vi "rqcAlice PM Level Test (Low Level Example).vi"() -> ()   [LabVIEW 2019]
uses:
  FPGA/Alice/Custom Controls/Main State Machine/rqcAlice DAC Clock Positions.ctl
  Shared/Shared FPGA Lib/Shared Logic/Custom Controls/rqc Random Generator.parameters.ctl
  Shared/Shared FPGA Lib/Shared Logic/Custom Controls/rqc Random Generator.value type.ctl
  FPGA/Alice/Custom Controls/Phase Modulator/rqcAlice Mod.Config.ctl
  Custom Controls/rqcAlice States.ctl
  Shared/Shared Host Lib/rqc ServiceNET/Custom Controls/rqc ServiceNET command.ctl
  Shared/Shared Host Lib/rqc ServiceNET/Alice/Custom Controls/rqcAlice ServiceNET control.ctl
  <vilib>/FPGAPlugInAG/PCIe-7820R/niLvFpga_Open_PCIe-7820R.vi
  <vilib>/rvi/interface/common/dynamic/niFpgaDynamicAddResources.vi
  <vilib>/FPGAPlugInAG/Dynamic/niLvFpga_Close_Dynamic.vi
  <vilib>/rvi/interface/nirviOpenFPGA/nirviOpenFPGA.xnode
  FPGA Bitfiles/rqcAlice FPGA (7820R) v 3.2.0.lvbitx
  <vilib>/rvi/interface/nirviCloseFPGA/nirviCloseFPGA.xnode
panel:
  in  "Tab Control":enum32{"Alice PM config", "Advanced parameters"}(tab)
  in  "Sync mode":bool caption="«Coax / SD»"
  in  "PM.DAC parameters":T1={"value type"=enum."constant", "constant"=512, "num of levels"=4, "levels values"=[512, 512, 512, 512]} caption="Phase modulation value" {"num of levels" min=4 max=4 step=1}
  in  "PM min":u16
  in  "PM max":u16=512
  in  "PM increment":u16=8
  out "PM value scanned":u16=512
  in  "Delay line value":u32
  in  "Modulator config":T3={"mod.on"=9, "mod.off"=1}
  in  "DAC Clock params":T4=[18, 38]
  out "IP Address":string="10.32.64.203"
  out "Num of Detections vs DAC Level":T5(graph)={"appended array"=[0.0, 8.0, 16.0, 24.0, 32.0, 40.0, 48.0, 56.0, 64.0, 72.0, 80.0, 88.0, 96.0, 104.0, 112.0, 120.0, 128.0, 136.0, 144.0, 152.0, 160.0, 168.0, 176.0, 184.0, 192.0, 200.0, 208.0, 216.0, 224.0, 232.0, 240.0, 248.0, 256.0, 264.0, 272.0, 280.0, 288.0, 296.0, 304.0, 312.0, 320.0, 328.0, 336.0, 344.0, 352.0, 360.0, 368.0, 376.0, 384.0, 392.0, 400.0, 408.0, 416.0, 424.0, 432.0, 440.0, 448.0, 456.0, 464.0, 472.0, 480.0, 488.0, 496.0, 504.0, 512.0, 512.0], "appended array"=[0.0, 0.0, 0.0, 0.0, 0.0, 0.0, 0.0, 0.0, 0.0, 0.0, 0.0, 0.0, 0.0, 0.0, 0.0, 0.0, 0.0, 0.0, 0.0, 0.0, 0.0, 0.0, 0.0, 0.0, 0.0, 0.0, 0.0, 0.0, 0.0, 0.0, 0.0, 0.0, 0.0, 0.0, 0.0, 0.0, 0.0, 0.0, 0.0, 0.0, 0.0, 0.0, 0.0, 0.0, 0.0, 0.0, 0.0, 0.0, 0.0, 0.0, 0.0, 0.0, 0.0, 0.0, 0.0, 0.0, 0.0, 0.0, 0.0, 0.0, 0.0, 0.0, 0.0, 0.0, 0.0]}
  out "error out":errorcluster
  in  "Stop":bool
  out "Connection status":bool
  in  "port":u16=5020
  out "Current State":T6=enum."App.Stop" caption="App current state"
  in  "Attenuation, dB":dbl=10.0 max=40.0
  # "LAN settings:"
  # "«"
  # "»"
  # "Constant"
  # "Random"
  # "Recommended [18]\n[38]"
  # "Recommended mod.on - [9]\nmod.off - [1-2]"
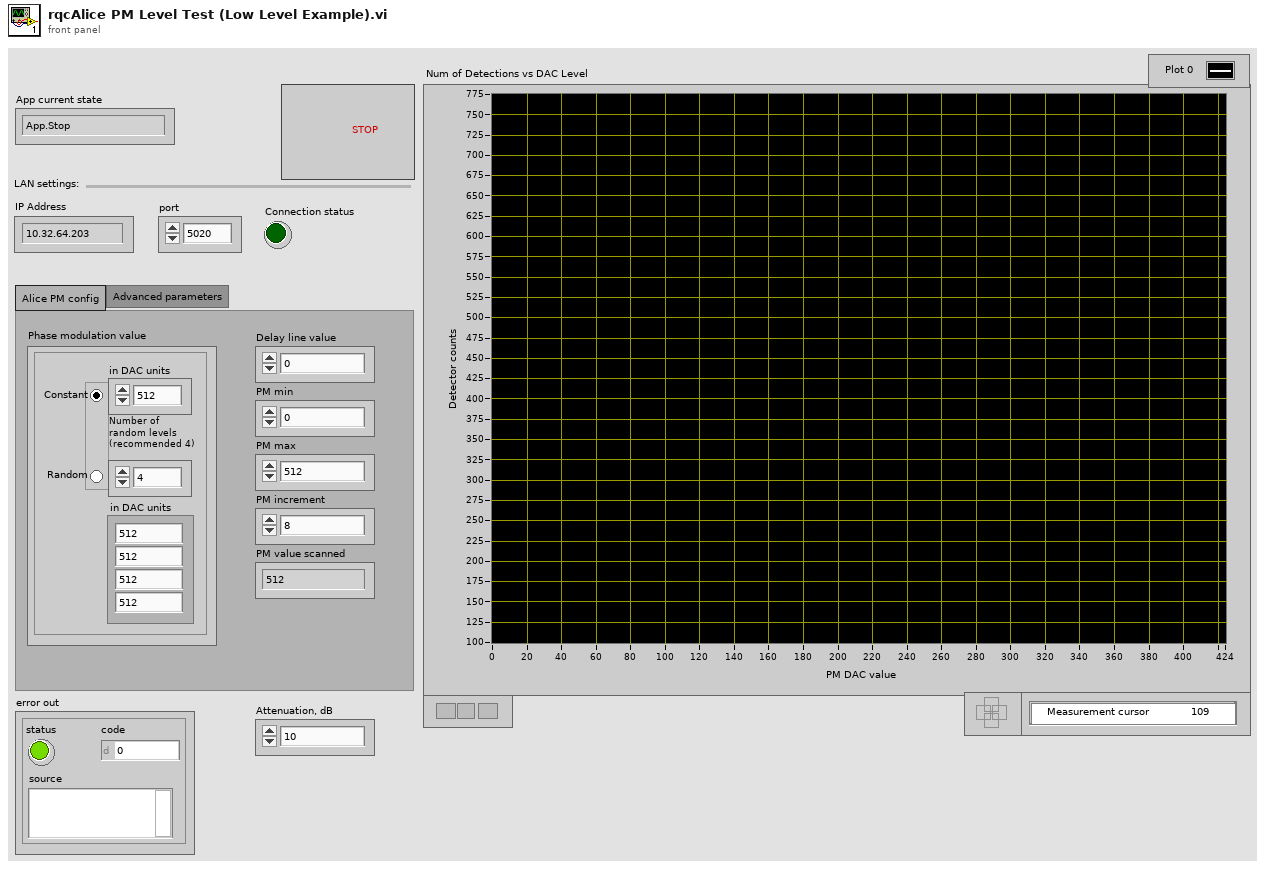
[diagram p1: front panel]
types:
  T1 = typedef "rqc Random Generator.parameters.ctl" = cluster{"value type":T2, "constant":u16, "num of levels":u16, "levels values":u16[]}
  T2 = typedef "rqc Random Generator.value type.ctl" = enum32{"random value", "constant"}
  T3 = typedef "rqcAlice Mod.Config.ctl" = cluster{"mod.on":u8, "mod.off":u8}
  T4 = typedef "rqcAlice DAC Clock Positions.ctl" = u8[]
  T5 = cluster{"appended array":dbl[], "appended array":dbl[]}
  T6 = typedef "rqcAlice States.ctl" = enum16{"HW.configure", "HW.meas", "NET.create", "NET.connect", "NET.readCommand", "NET.sendCommand", "NET.readData", "NET.close", "Meas.Start", "Meas.NextStep", "Meas.restart", "Meas.Done", "App.HandleEvent", "App.HandleError", "App.Stop"}
  T7 = typedef "rqc ServiceNET command.ctl" = enum8{"NONE", "READY", "START", "PING"}
  T8 = typedef "rqcAlice ServiceNET control.ctl" = cluster{"connection ID":refnum<k5>, "port":u16, "connected?":bool}
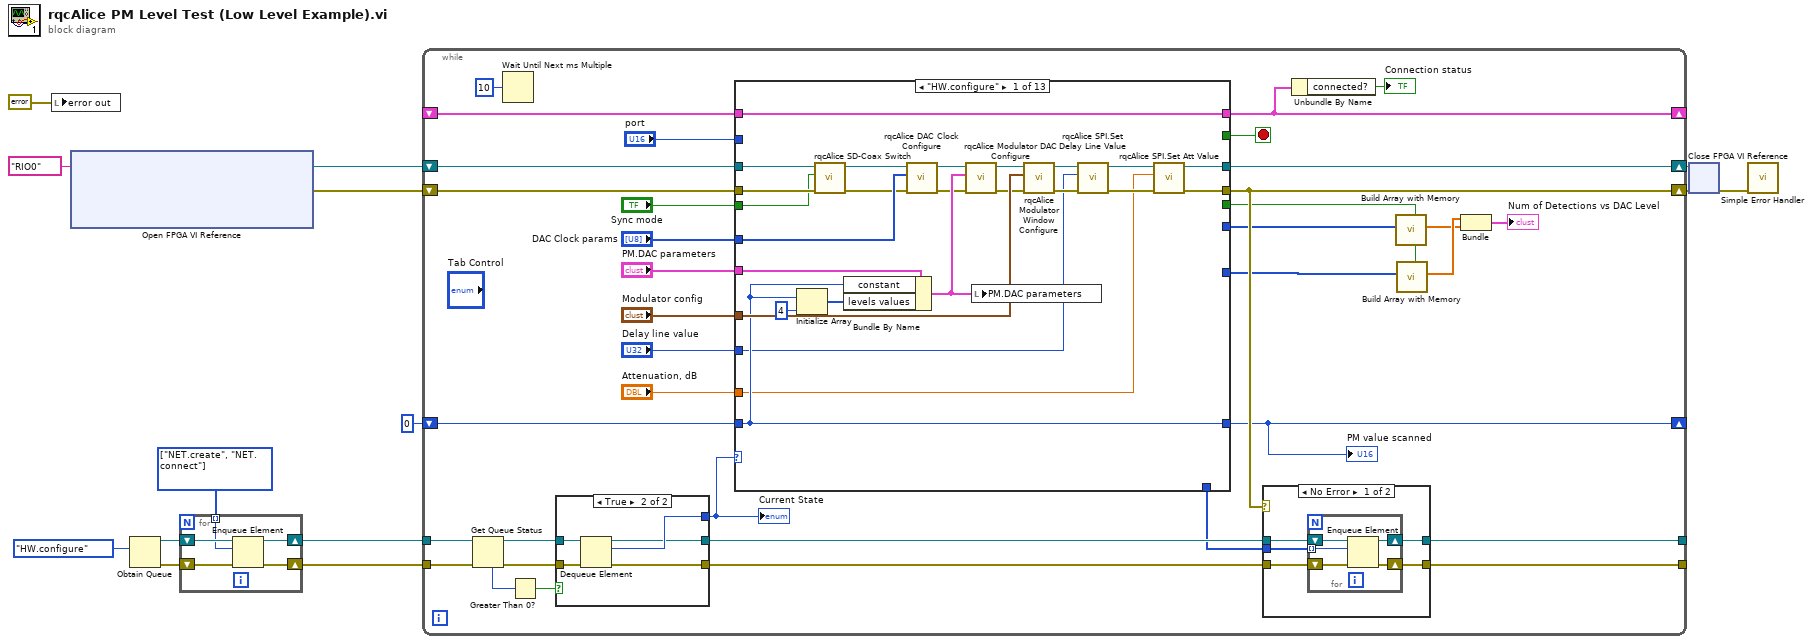
[diagram p0: block diagram]
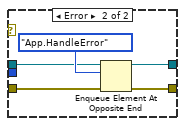
[diagram p2: hidden frame]
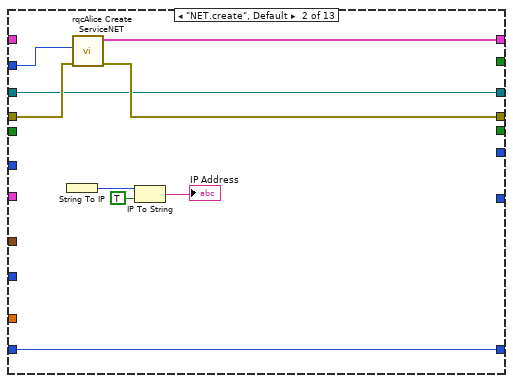
[diagram p3: hidden frame]
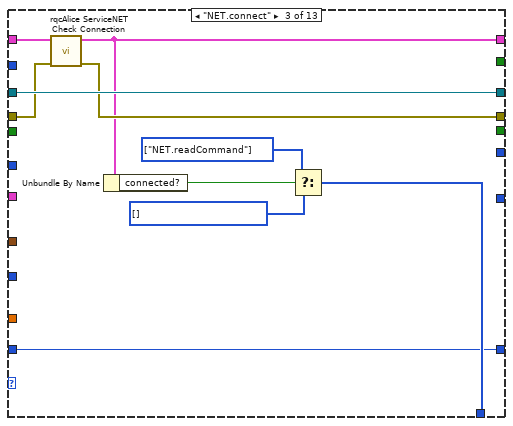
[diagram p4: hidden frame]
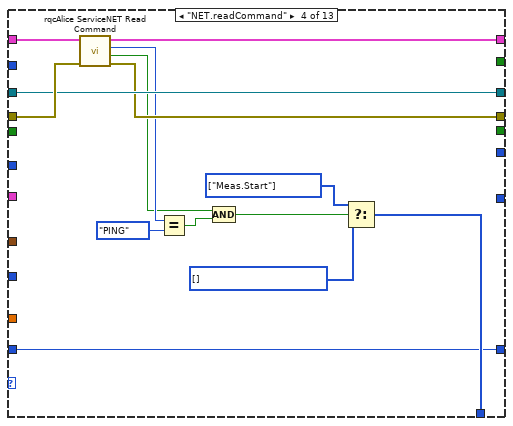
[diagram p5: hidden frame]
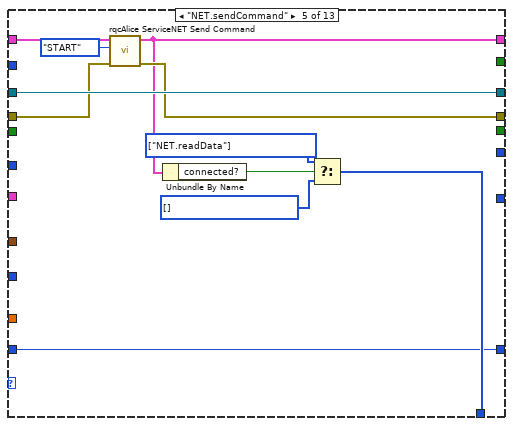
[diagram p6: hidden frame]
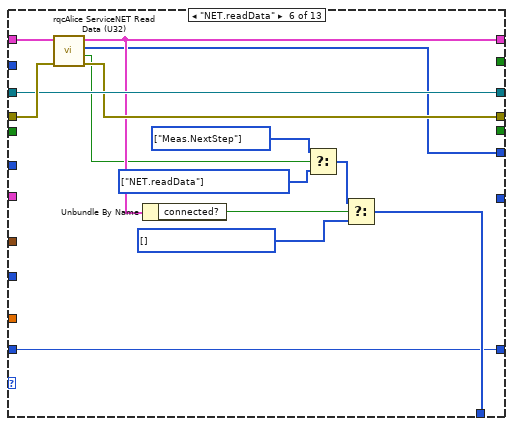
[diagram p7: hidden frame]
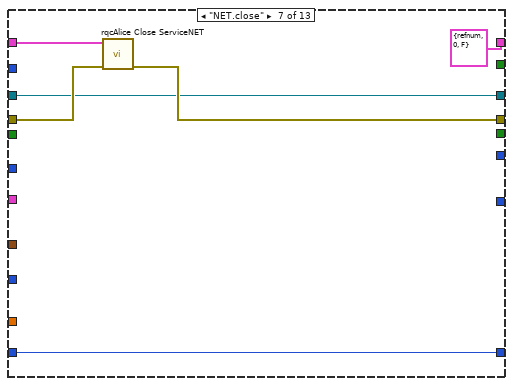
[diagram p8: hidden frame]
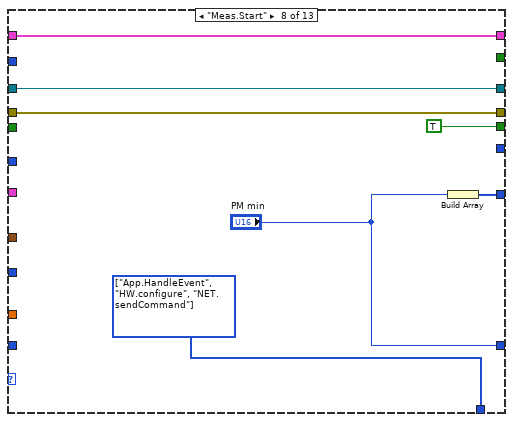
[diagram p9: hidden frame]
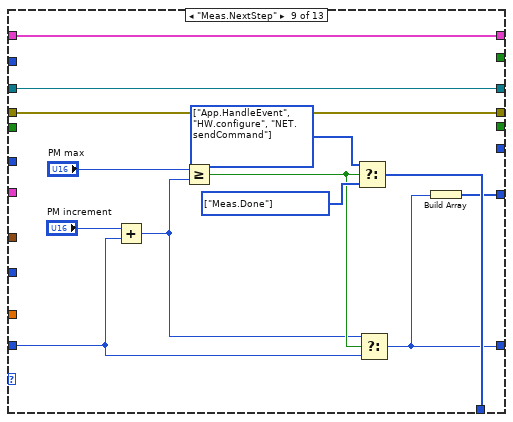
[diagram p10: hidden frame]
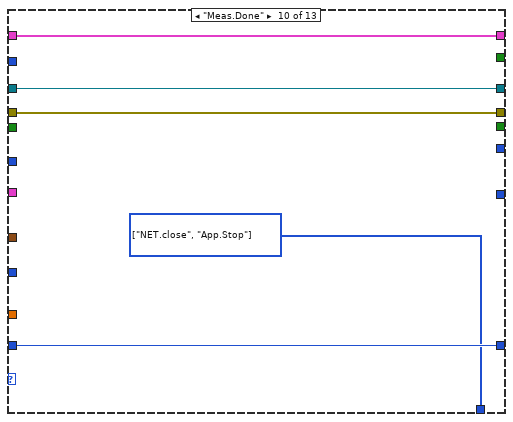
[diagram p11: hidden frame]
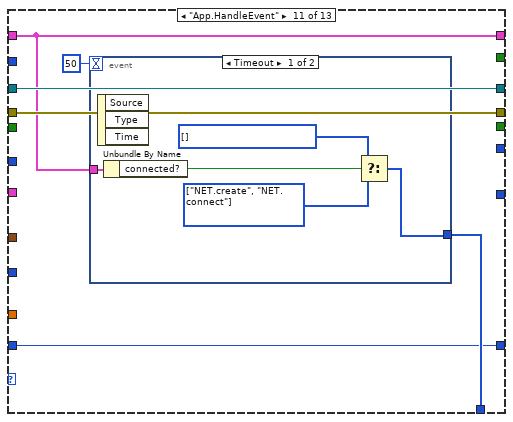
[diagram p12: hidden frame]
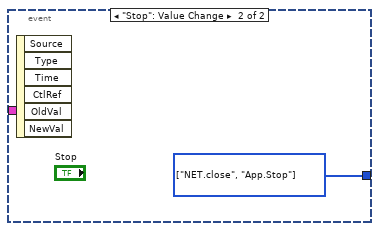
[diagram p13: hidden frame]
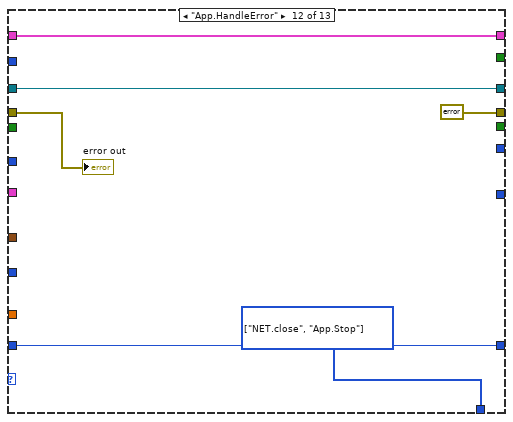
[diagram p14: hidden frame]
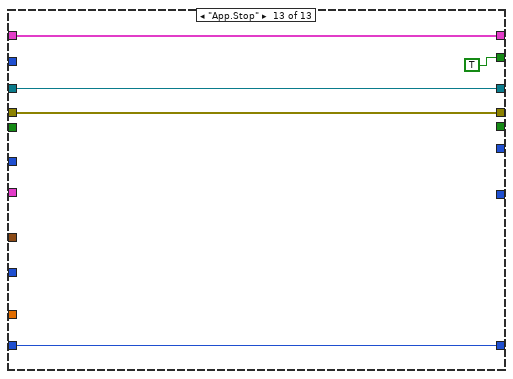
[diagram p15: hidden frame]
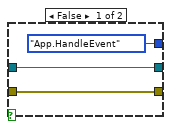
[diagram p16: hidden frame]
diagram:
  w6 = T6[] [enum."NET.create", enum."NET.connect"] items=["HW.configure", "HW.meas", "NET.create", "NET.connect", "NET.readCommand", "NET.sendCommand", "NET.readData", "NET.close", "Meas.Start", "Meas.NextStep", "Meas.restart", "Meas.Done", "App.HandleEvent", "App.HandleError", "App.Stop"]
  n1 = local write "error out"(errorcluster {"status"=FALSE, "code"=0, "source"=""} ("error out")) -> ()
  n2 = xnode "Open FPGA VI Reference"("resource name"=tag "RIO0") -> ("FPGA VI Reference Out"=w13:refnum<k20>, "error out"=w12:errorcluster)  [unwired: 1 in]
  n3 = Obtain Queue(element data type=rqcAlice_States."HW.configure" ("rqcAlice States")) -> (queue out=w8:refnum<queue>, error out=w7:errorcluster)  [unwired: 4 in, 1 out]
  n4 = for {
    shift-right: [w17] -> w5
    shift-left: w8 -> [w19]
    shift-right: [w16] -> w4
    shift-left: w7 -> [w18]
    tunnel: w6 -> [w15] mode=indexing
    n5 = Enqueue Element(queue=w19, element=w15, error in (no error)=w18) -> (queue out=w17:refnum<queue>, error out=w16:errorcluster)  [unwired: 1 in, 1 out]
  }
  n6 = while {
    tunnel: w5 -> [w49]
    shift-right: [w50] -> w11
    shift-left: w13 -> [w55]
    shift-right: [w42] -> w10
    shift-left: w12 -> [w53]
    tunnel: w4 -> [w48]
    tunnel: [w39] -> _
    tunnel: [w38] -> _
    shift-right: [w34] -> _
    shift-left: _ -> [w36]
    shift-right: [w28] -> _
    shift-left: u16 0 ("Delay Line min") -> [w30]
    stop <- w32 stop-if-true
    n7 = Get Queue Status(queue=w49, error in (no error)=w48) -> (queue out=w45:refnum<queue>, error out=w44:errorcluster, # elements in queue=w47:i32)  [unwired: 1 in, 5 out]
    n8 = Wait Until Next ms Multiple(millisecond multiple=u32 10) -> ()  [unwired: 1 out]
    n9 = Greater Than 0?(x=w47) -> (x > 0?=w46:bool)
    n10 = case shown="True" w46 {
      tunnel: w45 -> [w209 w215]
      tunnel: w44 -> [w208 w214]
      tunnel: [rqcAlice_States."App.HandleEvent" ("rqcAlice States") w213] -> w43
      tunnel: [w209 w212] -> w41
      tunnel: [w208 w211] -> w40
      frame False {
      }
      frame True {
        n11 = Dequeue Element(queue=w215, error in (no error)=w214) -> (queue out=w212:refnum<queue>, element=w213:T6, error out=w211:errorcluster)  [unwired: 1 in, 1 out]
      }
    }
    "Current State" <- w43
    n12 = case shown="\"HW.configure\"" w43 {
      tunnel: w55 -> [w75 w101 w114 w125 w139 w151 w155 w165 w178 w183 w190 w201 w206]
      tunnel: "DAC Clock params" -> [w95 _ _ _ _ _ _ _ _ _ _ _ _]
      tunnel: w53 -> [w73 w103 w112 w127 w137 w152 w158 w164 w177 w182 w189 w200 w205]
      tunnel: "PM.DAC parameters" -> [w92 _ _ _ _ _ _ _ _ _ _ _ _]
      tunnel: "Modulator config" -> [w94 _ _ _ _ _ _ _ _ _ _ _ _]
      tunnel: [w84 w101 w114 w125 w139 w151 w155 w165 w178 w183 w190 w201 w206] -> w50
      tunnel: [w82 w102 w111 w124 w136 w150 w157 w164 w177 w182 w189 errorcluster {"status"=FALSE, "code"=0, "source"=""} ("error out") w205] -> w42
      tunnel: [_ _ w107 w116 w130 w142 _ w163 w173 w180 w186 w198 _] -> w37
      tunnel: [w93 w104 w110 w126 w134 w149 T8 {"connection ID"=refnum, "port"=0, "connected?"=FALSE} ("rqcAlice ServiceNET out") w166 w179 w184 w187 w202 w204] -> w34
      tunnel: w36 -> [w93 _ w113 w128 w138 w153 w159 w166 w179 w184 w187 w202 w204]
      tunnel: "port" -> [_ w100 _ _ _ _ _ _ _ _ _ _ _]
      tunnel: [_ _ _ _ _ _ _ _ _ _ _ _ TRUE] -> w32
      tunnel: w30 -> [w89 w99 w105 w115 w129 w141 w154 _ w169 w181 w185 w197 w203]
      tunnel: [w89 w99 w105 w115 w129 w141 w154 "PM min" w168 w181 w185 w197 w203] -> w28
      tunnel: [_ _ _ _ _ w140 _ _ _ _ _ _ _] -> w29
      tunnel: [_ _ _ _ _ _ _ w160 w167 _ _ _ _] -> w27
      tunnel: [_ _ _ _ _ _ _ TRUE _ _ _ _ _] -> w26
      tunnel: "Delay line value" -> [w86 _ _ _ _ _ _ _ _ _ _ _ _]
      tunnel: "Attenuation, dB" -> [w81 _ _ _ _ _ _ _ _ _ _ _ _]
      tunnel: "Sync mode" -> [w71 _ _ _ _ _ _ _ _ _ _ _ _]
      frame "HW.configure" {
        n13 = Initialize Array(w89, 4 ("dimension size")) -> (w90:u16[])
        n14 = call "rqcAlice SD-Coax Switch.vi"("error in"=w73, "SD/Coax Select"=w71, "Alice FPGA Reference In"=w75) -> ("error out"=w72:errorcluster, "Alice FPGA Reference Out"=w74:refnum<k20>)  [unwired: 7 in]
        n15 = Bundle By Name(cluster=w92, "constant"=w89, "levels values"=w90) -> (w79:T1)
        n16 = call "rqcAlice DAC Clock Configure.vi"("error in"=w72, "DAC Clock params"=w95, "Alice FPGA Reference In"=w74) -> ("error out"=w78:errorcluster, "Alice FPGA Reference Out"=w80:refnum<k20>)  [unwired: 7 in]
        n17 = call "rqcAlice Modulator DAC Configure.vi"("error in"=w78, "RndGen.parameters"=w79, "Alice FPGA Reference In"=w80) -> ("error out"=w77:errorcluster, "Alice FPGA Reference Out"=w76:refnum<k20>)  [unwired: 7 in]
        n18 = local write "PM.DAC parameters"(w79) -> ()
        n19 = call "rqcAlice Modulator Window Configure.vi"("error in"=w77, "Modulator config"=w94, "Alice FPGA Reference In"=w76) -> ("error out"=w88:errorcluster, "Alice FPGA Reference Out"=w87:refnum<k20>)  [unwired: 7 in]
        n20 = call "rqcAlice SPI.Set Delay Line Value.vi"("error in"=w88, "Delay Line Value"=w86, "Alice FPGA Reference In"=w87) -> ("error out"=w83:errorcluster, "Alice FPGA Reference Out"=w85:refnum<k20>)  [unwired: 7 in]
        n21 = call "rqcAlice SPI.Set Att Value.vi"("error in"=w83, "Attenuation, dB"=w81, "Alice FPGA Reference In"=w85) -> ("error out"=w82:errorcluster, "Alice FPGA Reference Out"=w84:refnum<k20>)  [unwired: 7 in]
      }
      frame "NET.create", Default {
        n22 = String To IP() -> (0:w97:u32)  [unwired: 1 in]
        n23 = call "rqcAlice Create ServiceNET.vi"("error in"=w103, "port"=w100) -> ("error out"=w102:errorcluster, "rqcAlice ServiceNET control"=w104:T8)  [unwired: 8 in]
        n24 = IP To String(1:TRUE ("dot notation? (F)"), 2:w97) -> (0:→"IP Address":string)
      }
      frame "NET.connect" {
        w106 = T6[] [] items=["HW.configure", "HW.meas", "NET.create", "NET.connect", "NET.readCommand", "NET.sendCommand", "NET.readData", "NET.close", "Meas.Start", "Meas.NextStep", "Meas.restart", "Meas.Done", "App.HandleEvent", "App.HandleError", "App.Stop"] ("f")
        w108 = T6[] [enum."NET.readCommand"] items=["HW.configure", "HW.meas", "NET.create", "NET.connect", "NET.readCommand", "NET.sendCommand", "NET.readData", "NET.close", "Meas.Start", "Meas.NextStep", "Meas.restart", "Meas.Done", "App.HandleEvent", "App.HandleError", "App.Stop"]
        n25 = call "rqcAlice ServiceNET Check Connection.vi"("error in"=w112, "rqcAlice ServiceNET in"=w113) -> ("error out"=w111:errorcluster, "rqcAlice ServiceNET out"=w110:T8)  [unwired: 8 in]
        n26 = Unbundle By Name(w110) -> ("connected?"=w109:bool)
        n27 = Select(t=w108, s=w109, f=w106) -> (s? t:f=w107:T6[])
      }
      frame "NET.readCommand" {
        w117 = T6[] [] items=["HW.configure", "HW.meas", "NET.create", "NET.connect", "NET.readCommand", "NET.sendCommand", "NET.readData", "NET.close", "Meas.Start", "Meas.NextStep", "Meas.restart", "Meas.Done", "App.HandleEvent", "App.HandleError", "App.Stop"] ("f")
        w118 = T6[] [enum."Meas.Start"] items=["HW.configure", "HW.meas", "NET.create", "NET.connect", "NET.readCommand", "NET.sendCommand", "NET.readData", "NET.close", "Meas.Start", "Meas.NextStep", "Meas.restart", "Meas.Done", "App.HandleEvent", "App.HandleError", "App.Stop"] ("f")
        n28 = call "rqcAlice ServiceNET Read Command.vi"("error in"=w127, "rqcAlice ServiceNET in"=w128) -> ("error out"=w124:errorcluster, "cmd valid"=w120:bool, "command"=w122:T7, "rqcAlice ServiceNET out"=w126:T8)  [unwired: 6 in]
        n29 = Equal?(x=w122, y=rqc_ServiceNET_command."PING" ("command")) -> (x = y?=w121:bool)
        n30 = Compound Arithmetic op=AND(w120, w121) -> (w119:bool)
        n31 = Select(t=w118, s=w119, f=w117) -> (s? t:f=w116:T6[])
      }
      frame "NET.sendCommand" {
        w131 = T6[] [] items=["HW.configure", "HW.meas", "NET.create", "NET.connect", "NET.readCommand", "NET.sendCommand", "NET.readData", "NET.close", "Meas.Start", "Meas.NextStep", "Meas.restart", "Meas.Done", "App.HandleEvent", "App.HandleError", "App.Stop"] ("f")
        w132 = T6[] [enum."NET.readData"] items=["HW.configure", "HW.meas", "NET.create", "NET.connect", "NET.readCommand", "NET.sendCommand", "NET.readData", "NET.close", "Meas.Start", "Meas.NextStep", "Meas.restart", "Meas.Done", "App.HandleEvent", "App.HandleError", "App.Stop"] ("f")
        n32 = call "rqcAlice ServiceNET Send Command.vi"("error in"=w137, "command"=rqc_ServiceNET_command."START", "rqcAlice ServiceNET in"=w138) -> ("error out"=w136:errorcluster, "rqcAlice ServiceNET out"=w134:T8)  [unwired: 7 in]
        n33 = Unbundle By Name(w134) -> ("connected?"=w133:bool)
        n34 = Select(t=w132, s=w133, f=w131) -> (s? t:f=w130:T6[])
      }
      frame "NET.readData" {
        w143 = T6[] [] items=["HW.configure", "HW.meas", "NET.create", "NET.connect", "NET.readCommand", "NET.sendCommand", "NET.readData", "NET.close", "Meas.Start", "Meas.NextStep", "Meas.restart", "Meas.Done", "App.HandleEvent", "App.HandleError", "App.Stop"] ("f")
        w148 = T6[] [enum."Meas.NextStep"] items=["HW.configure", "HW.meas", "NET.create", "NET.connect", "NET.readCommand", "NET.sendCommand", "NET.readData", "NET.close", "Meas.Start", "Meas.NextStep", "Meas.restart", "Meas.Done", "App.HandleEvent", "App.HandleError", "App.Stop"] ("t")
        w146 = T6[] [enum."NET.readData"] items=["HW.configure", "HW.meas", "NET.create", "NET.connect", "NET.readCommand", "NET.sendCommand", "NET.readData", "NET.close", "Meas.Start", "Meas.NextStep", "Meas.restart", "Meas.Done", "App.HandleEvent", "App.HandleError", "App.Stop"] ("f")
        n35 = call "rqcAlice ServiceNET Read Data (U32).vi"("error in"=w152, "rqcAlice ServiceNET in"=w153) -> ("error out"=w150:errorcluster, "data valid"=w147:bool, "data"=w140:u32[], "rqcAlice ServiceNET out"=w149:T8)  [unwired: 6 in]
        n36 = Unbundle By Name(w149) -> ("connected?"=w145:bool)
        n37 = Select(t=w148, s=w147, f=w146) -> (s? t:f=w144:T6[])
        n38 = Select(t=w144, s=w145, f=w143) -> (s? t:f=w142:T6[])
      }
      frame "NET.close" {
        n39 = call "rqcAlice Close ServiceNET.vi"("error in"=w158, "rqcAlice ServiceNET in"=w159) -> ("error out"=w157:errorcluster)  [unwired: 9 in]
      }
      frame "Meas.Start" {
        w163 = T6[] [enum."App.HandleEvent", enum."HW.configure", enum."NET.sendCommand"] items=["HW.configure", "HW.meas", "NET.create", "NET.connect", "NET.readCommand", "NET.sendCommand", "NET.readData", "NET.close", "Meas.Start", "Meas.NextStep", "Meas.restart", "Meas.Done", "App.HandleEvent", "App.HandleError", "App.Stop"] ("f")
        n40 = Build Array("PM min") -> (w160:u16[])
      }
      frame "Meas.NextStep" {
        w172 = T6[] [enum."Meas.Done"] items=["HW.configure", "HW.meas", "NET.create", "NET.connect", "NET.readCommand", "NET.sendCommand", "NET.readData", "NET.close", "Meas.Start", "Meas.NextStep", "Meas.restart", "Meas.Done", "App.HandleEvent", "App.HandleError", "App.Stop"] ("f")
        w174 = T6[] [enum."App.HandleEvent", enum."HW.configure", enum."NET.sendCommand"] items=["HW.configure", "HW.meas", "NET.create", "NET.connect", "NET.readCommand", "NET.sendCommand", "NET.readData", "NET.close", "Meas.Start", "Meas.NextStep", "Meas.restart", "Meas.Done", "App.HandleEvent", "App.HandleError", "App.Stop"] ("f")
        n41 = Add(x="PM increment", y=w169) -> (x+y=w170:u16)
        n42 = Greater Or Equal?(x="PM max", y=w170) -> (x >= y?=w171:bool)
        n43 = Select(t=w174, s=w171, f=w172) -> (s? t:f=w173:T6[])
        n44 = Select(t=w170, s=w171, f=w169) -> (s? t:f=w168:u16)
        n45 = Build Array(w168) -> (w167:u16[])
      }
      frame "Meas.Done" {
        w180 = T6[] [enum."NET.close", enum."App.Stop"] items=["HW.configure", "HW.meas", "NET.create", "NET.connect", "NET.readCommand", "NET.sendCommand", "NET.readData", "NET.close", "Meas.Start", "Meas.NextStep", "Meas.restart", "Meas.Done", "App.HandleEvent", "App.HandleError", "App.Stop"] ("f")
      }
      frame "App.HandleEvent" {
        n46 = event shown="[0] Timeout" {
          selector: _ -> [_ _]
          dyn-events: _ -> [_ _]
          timeout: 50 -> [_ _]
          tunnel: w187 -> [w195 _]
          tunnel: [w191 w196] -> w186
          event Timeout {
            w192 = T6[] [enum."NET.create", enum."NET.connect"] items=["HW.configure", "HW.meas", "NET.create", "NET.connect", "NET.readCommand", "NET.sendCommand", "NET.readData", "NET.close", "Meas.Start", "Meas.NextStep", "Meas.restart", "Meas.Done", "App.HandleEvent", "App.HandleError", "App.Stop"]
            w193 = T6[] [] items=["HW.configure", "HW.meas", "NET.create", "NET.connect", "NET.readCommand", "NET.sendCommand", "NET.readData", "NET.close", "Meas.Start", "Meas.NextStep", "Meas.restart", "Meas.Done", "App.HandleEvent", "App.HandleError", "App.Stop"]
            n47 = event-data() -> ()  [unwired: 1 in, 3 out]
            n48 = Unbundle By Name(w195) -> ("connected?"=w194:bool)
            n49 = Select(t=w193, s=w194, f=w192) -> (s? t:f=w191:T6[])
          }
          event "Stop": Value Change {
            w196 = T6[] [enum."NET.close", enum."App.Stop"] items=["HW.configure", "HW.meas", "NET.create", "NET.connect", "NET.readCommand", "NET.sendCommand", "NET.readData", "NET.close", "Meas.Start", "Meas.NextStep", "Meas.restart", "Meas.Done", "App.HandleEvent", "App.HandleError", "App.Stop"]
            n50 = event-data() -> ()  [unwired: 1 in, 6 out]
          }
        }
      }
      frame "App.HandleError" {
        w198 = T6[] [enum."NET.close", enum."App.Stop"] items=["HW.configure", "HW.meas", "NET.create", "NET.connect", "NET.readCommand", "NET.sendCommand", "NET.readData", "NET.close", "Meas.Start", "Meas.NextStep", "Meas.restart", "Meas.Done", "App.HandleEvent", "App.HandleError", "App.Stop"] ("f")
        "error out" <- w200
      }
      frame "App.Stop" {
      }
    }
    "PM value scanned" <- w28
    n51 = case shown="No Error" w42 {
      tunnel: w41 -> [w60 w69]
      tunnel: w40 -> [w59 w67]
      tunnel: [w58 w68] -> w39
      tunnel: [w57 w66] -> w38
      tunnel: w37 -> [w56 _]
      frame No Error {
        n52 = for {
          shift-right: [w63] -> w58
          shift-left: w60 -> [w65]
          shift-right: [w62] -> w57
          shift-left: w59 -> [w64]
          tunnel: w56 -> [w61] mode=indexing
          n53 = Enqueue Element(queue=w65, element=w61, error in (no error)=w64) -> (queue out=w63:refnum<queue>, error out=w62:errorcluster)  [unwired: 1 in, 1 out]
        }
      }
      frame Error {
        n54 = Enqueue Element At Opposite End(queue=w69, element=rqcAlice_States."App.HandleError" ("rqcAlice States"), error in (no error)=w67) -> (queue out=w68:refnum<queue>, error out=w66:errorcluster)  [unwired: 1 in, 1 out]
      }
    }
    n55 = Unbundle By Name(w34) -> ("connected?"=→"Connection status":bool)
    n56 = call "Build Array with Memory.vi"("reset"=w26, "new array"=w29) -> ("appended array"=w23:dbl[])  [unwired: 9 in]
    n57 = call "Build Array with Memory.vi"("reset"=w26, "new array"=w27) -> ("appended array"=w24:dbl[])  [unwired: 9 in]
    n58 = Bundle("appended array"=w24, "appended array"=w23) -> (→"Num of Detections vs DAC Level":T5)  [unwired: 1 in]
  }
  n59 = xnode "Close FPGA VI Reference"("FPGA VI Reference In"=w11, "error in"=w10) -> ("error out"=w3:errorcluster)
  n60 = call <vilib>:"Simple Error Handler.vi"("error in (no error)"=w3) -> ()  [unwired: 4 in, 5 out]
